vi "For Loop Sine Wave.vi"() -> ()   [LabVIEW 2017]
panel:
  out "Graph - Stored Data":dbl[](graph)
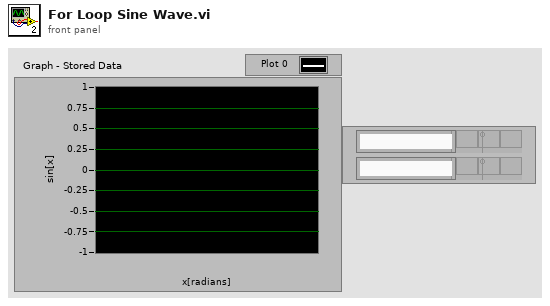
[diagram p1: front panel]
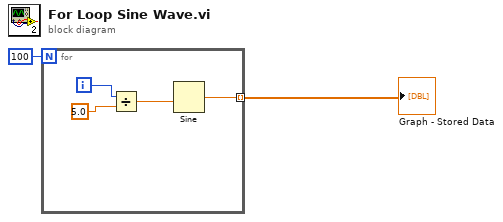
[diagram p0: block diagram]
diagram:
  n1 = for {
    N: 100 -> [_]
    tunnel: [w3] -> w1 mode=indexing
    i -> [w5]
    n2 = Divide(x=w5, y=5.0) -> (x/y=w4:dbl)
    n3 = Sine(x=w4) -> (sin(x)=w3:dbl)
  }
  "Graph - Stored Data" <- w1
